vi "PING))) demo(not).vi"() -> ()   [LabVIEW 2016]
uses:
  <vilib>/myRIO/Instrument Drivers/Onboard IO/DIO/typedefs/DIO Reference.ctl
  <vilib>/myRIO/Common/Instrument Driver Framework/Utilities/typedefs/myRIO Generic Hardware Reference.ctl
  <vilib>/myRIO/Common/Instrument Driver Framework/Utilities/typedefs/Hardware Version Enum.ctl
  <vilib>/myRIO/Common/Instrument Driver Framework/Utilities/typedefs/myRIO v1.0 Reference.ctl
  <vilib>/myRIO/Common/Instrument Driver Framework/Utilities/typedefs/Generic FPGA Reference.ctl
  <vilib>/myRIO/Common/Instrument Driver Framework/myRIO v1.0/DIO/typedefs/DIO Channels List.ctl
  <vilib>/myRIO/Common/Instrument Driver Framework/myRIO v1.0/DIO/typedefs/DIO Channels Enum.ctl
  <vilib>/myRIO/Common/Instrument Driver Framework/myRIO v1.0/DIO/vis/myRIO v1.0 Close DIO.vi
  <vilib>/myRIO/Common/Instrument Driver Framework/myRIO v1.0/DIO/vis/myRIO v1.0 Unreserve DIO.vi
  <vilib>/myRIO/Common/Instrument Driver Framework/myRIO v1.0/DIO/vis/myRIO v1.0 Build MUX Configuration DIO.vi
  <vilib>/myRIO/Common/Instrument Driver Framework/myRIO v1.0/Resource Manager/vis/myRIO v1.0 Unreserve Channel List.vi
  <vilib>/myRIO/Common/Instrument Driver Framework/myRIO v1.0/Resource Manager/vis/myRIO v1.0 Create Configuration List.vi
  <vilib>/myRIO/Common/Instrument Driver Framework/myRIO v1.0/Resource Manager/vis/myRIO v1.0 Unreserve Channel.vi
  <vilib>/myRIO/Common/Instrument Driver Framework/myRIO v1.0/Resource Manager/vis/myRIO v1.0 Build Mutex Name.vi
  <vilib>/Utility/error.llb/Error Cluster From Error Code.vi
  <vilib>/myRIO/Common/Instrument Driver Framework/myRIO v1.0/DIO/vis/myRIO v1.0 Write DIO.vi
  <vilib>/myRIO/Common/Instrument Driver Framework/myRIO v1.0/DIO/vis/myRIO v1.0 Read DIO.vi
  <vilib>/myRIO/Common/Instrument Driver Framework/myRIO v1.0/DIO/vis/myRIO v1.0 Shutdown DIO.vi
  <vilib>/myRIO/Common/Instrument Driver Framework/myRIO v1.0/Resource Manager/vis/myRIO v1.0 Configure IO.vi
  <vilib>/myRIO/Common/Instrument Driver Framework/Utilities/vis/Configuration Manager.vi
  <vilib>/myRIO/Common/Instrument Driver Framework/Utilities/vis/IO Manager.vi
  <vilib>/myRIO/Common/Instrument Driver Framework/myRIO v1.0/myRIO v1.0 Close.vi
  <vilib>/myRIO/Instrument Drivers/Onboard IO/DIO/DIO.lvlib
panel:
  out "distance":u32
  in  "Channel Names":tag[](array[tag])
  out "Enum":T1(ring)
  in  "error in (no error)":errorcluster
  in  "stop":bool
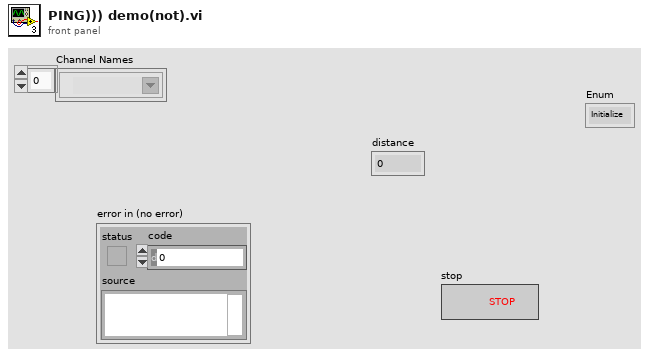
[diagram p1: front panel]
types:
  T1 = enum16{"Initialize", "Trigger pulse", "Wait pulse 1", "Wait pulse 2", "Calculate", "Stop"}
  T2 = typedef "DIO.lvlib/DIO Reference.ctl" = cluster{"myRIO Reference":T3, "DIO Channels List":T7}
  T3 = typedef "myRIO Generic Hardware Reference.ctl" = cluster{"myRIO Model":T4, "myRIO Hardware Reference":T5}
  T4 = typedef "Hardware Version Enum.ctl" = enum16{"Unknown", "myRIO-1900", "myRIO-1950", "roboRIO", "NI ELVIS RIO CM"}
  T5 = typedef "myRIO v1.0 Reference.ctl" = cluster{"Generic FPGA Reference":T6, "Allow multiple opens":bool}
  T6 = typedef "Generic FPGA Reference.ctl" = refnum<k20>
  T7 = typedef "DIO Channels List.ctl" = T8[]
  T8 = typedef "DIO Channels Enum.ctl" = enum16{"Not Connected", "C/DIO0", "C/DIO1", "C/DIO2", "C/DIO3", "C/DIO4", "C/DIO5", "C/DIO6", "C/DIO7", "A/DIO0", "A/DIO1", "A/DIO2", "A/DIO3", "A/DIO4", "A/DIO5", "A/DIO6", "A/DIO7", "A/DIO8", "A/DIO9", "A/DIO10", "A/DIO11", "A/DIO12", "A/DIO13", "A/DIO14", "A/DIO15", "B/DIO0", "B/DIO1", "B/DIO2", "B/DIO3", "B/DIO4", "B/DIO5", "B/DIO6", "B/DIO7", "B/DIO8", "B/DIO9", "B/DIO10", "B/DIO11", "B/DIO12", "B/DIO13", "B/DIO14", "B/DIO15", "LED0", "LED1", "LED2", "LED3", "Button0", "DIO/DIO0", "DIO/DIO1", "DIO/DIO2", "DIO/DIO3", "DIO/DIO4", "DIO/DIO5", "DIO/DIO6", "DIO/DIO7", "DIO/DIO8", "DIO/DIO9", "SPI/CS0", "SPI/CS1", "SPI/CS2", "SPI/CS3", "LED RADIO (Green)", "LED RADIO (Red)", "LED COMM (Green)", "LED COMM (Red)", "LED MODE (Green)", "LED MODE (Red)"}
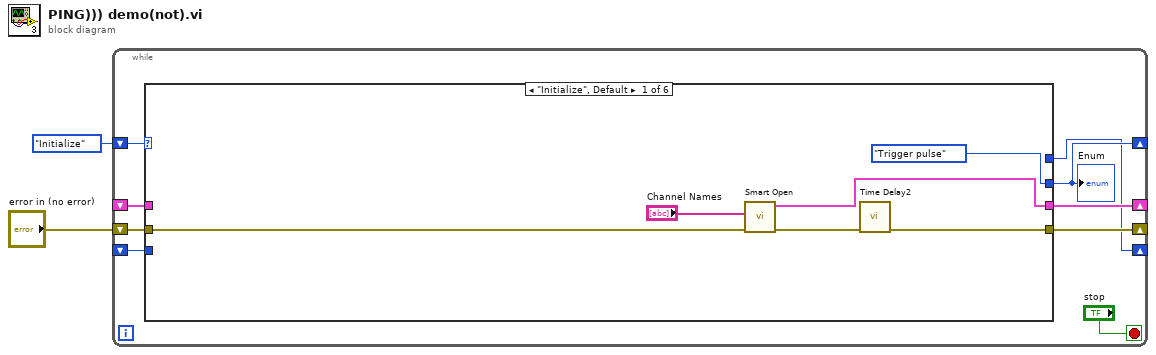
[diagram p0: block diagram]
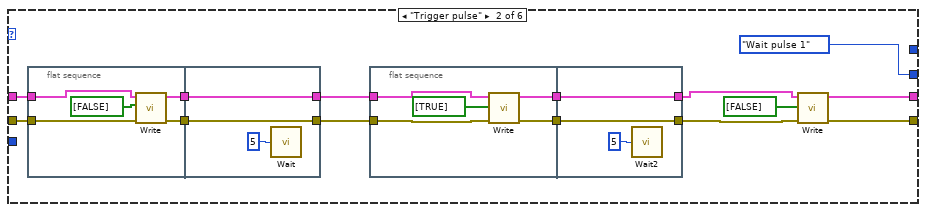
[diagram p2: hidden frame]
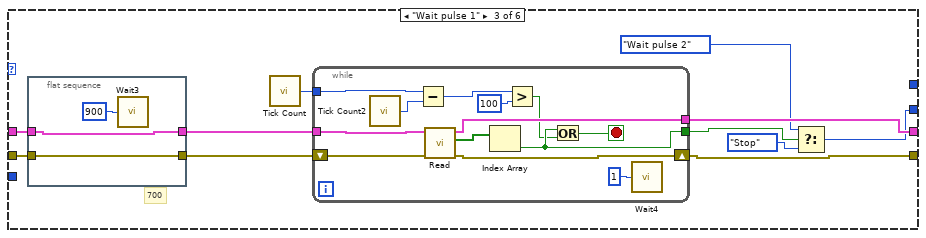
[diagram p3: hidden frame]
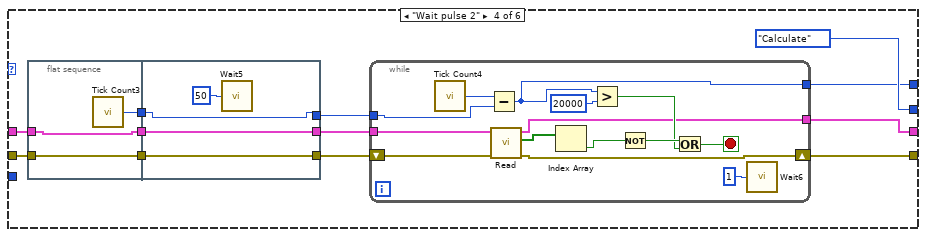
[diagram p4: hidden frame]
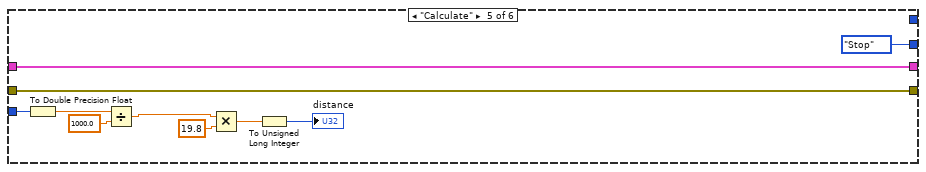
[diagram p5: hidden frame]
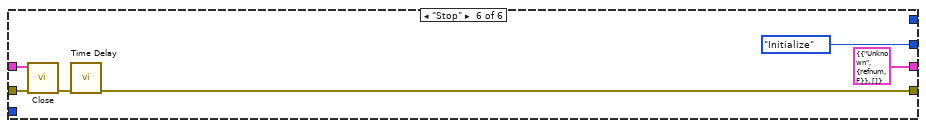
[diagram p6: hidden frame]
diagram:
  n1 = while {
    shift-right: [w9] -> _
    shift-left: T1."Initialize" -> [w10]
    shift-right: [w7] -> _
    shift-left: _ -> [w6]
    shift-right: [w5] -> _
    shift-left: "error in (no error)" -> [w8]
    shift-right: [w3] -> _
    shift-left: _ -> [w4]
    stop <- "stop" stop-if-true
    n2 = case shown="\"Initialize\", Default" w10 {
      tunnel: [T1."Trigger pulse" T1."Wait pulse 1" w49 T1."Calculate" T1."Stop" T1."Initialize"] -> w9
      tunnel: w8 -> [w16 w29 w57 w78 w112 w121]
      tunnel: [w15 w19 w54 w75 w113 T2 {"myRIO Reference"={"myRIO Model"=enum."Unknown", "myRIO Hardware Reference"={"Generic FPGA Reference"=refnum, "Allow multiple opens"=FALSE}}, "DIO Channels List"=[]} ("DIO Ref Out")] -> w7
      tunnel: w6 -> [_ w26 w55 w81 w113 w122]
      tunnel: [w12 w18 w53 w76 w112 w118] -> w5
      tunnel: w4 -> [_ _ _ _ w114 _]
      tunnel: [_ _ _ w77 _ _] -> w3
      frame "Initialize", Default {
        n3 = call <vilib>:"Smart Open.vi"("error in (no error)"=w16, "Channel Names"="Channel Names") -> ("error out"=w14:errorcluster, "DIO Ref Out"=w15:T2)  [unwired: 8 in]
        n4 = call "Time Delay2"("error in (no error)"=w14) -> ("error out"=w12:errorcluster)  [unwired: 10 in]
      }
      frame "Trigger pulse" {
        n5 = flat-sequence {
          tunnel: w29 -> [w43]
          tunnel: [w42] -> w27
          tunnel: w26 -> [w41]
          tunnel: [w40] -> w24
          tunnel: [w46] -> w28
          tunnel: w27 -> [w46]
          tunnel: [w45] -> w25
          tunnel: w24 -> [w45]
          frame #0 {
            n6 = call <vilib>:"Write.vi"("error in (no error)"=w43, "Values"=bool[] [FALSE], "DIO Ref In"=w41) -> ("error out"=w42:errorcluster, "DIO Ref Out"=w40:T2)  [unwired: 6 in]
          }
          frame #1 {
            n7 = call "Wait"("Count(uSec)"=u32 5) -> ()  [unwired: 1 out]
          }
        }
        n8 = flat-sequence {
          tunnel: w28 -> [w35]
          tunnel: w25 -> [w34]
          tunnel: [w33] -> w23
          tunnel: [w32] -> w21
          tunnel: w23 -> [w38]
          tunnel: [w38] -> w22
          tunnel: w21 -> [w37]
          tunnel: [w37] -> w20
          frame #0 {
            n9 = call <vilib>:"Write.vi"("error in (no error)"=w35, "Values"=bool[] [TRUE], "DIO Ref In"=w34) -> ("error out"=w32:errorcluster, "DIO Ref Out"=w33:T2)  [unwired: 6 in]
          }
          frame #1 {
            n10 = call "Wait2"("Count(uSec)"=u32 5) -> ()  [unwired: 1 out]
          }
        }
        n11 = call <vilib>:"Write.vi"("error in (no error)"=w20, "Values"=bool[] [FALSE], "DIO Ref In"=w22) -> ("error out"=w18:errorcluster, "DIO Ref Out"=w19:T2)  [unwired: 6 in]
      }
      frame "Wait pulse 1" {
        # "700"
        n12 = flat-sequence {
          tunnel: [w73] -> w58
          tunnel: w57 -> [w73]
          tunnel: [w72] -> w56
          tunnel: w55 -> [w72]
          frame #0 {
            n13 = call "Wait3"("Count(uSec)"=u32 900) -> ()  [unwired: 1 out]
          }
        }
        n14 = call "Tick Count"() -> ("Tick Count(uSec)"=w52:u32)
        n15 = while {
          tunnel: w56 -> [w70]
          tunnel: [w69] -> w54
          shift-right: [w66] -> w53
          shift-left: w58 -> [w71]
          tunnel: w52 -> [w61]
          tunnel: [w60] -> w48
          stop <- w67 stop-if-true
          n16 = call "Tick Count2"() -> ("Tick Count(uSec)"=w62:u32)
          n17 = Subtract(x=w61, y=w62) -> (x-y=w63:u32)
          n18 = call <vilib>:"Read.vi"("error in (no error)"=w71, "DIO Ref In"=w70) -> ("error out"=w66:errorcluster, "Values"=w68:bool[], "DIO Ref Out"=w69:T2)  [unwired: 7 in]
          n19 = Index Array(array=w68) -> (element=w60:bool)  [unwired: 1 in]
          n20 = Greater?(x=w63, y=u32 100) -> (0:w59:bool)
          n21 = Or(x=w60, y=w59) -> (x .or. y?=w67:bool)
          n22 = call "Wait4"("Count(uSec)"=u32 1) -> ()  [unwired: 1 out]
        }
        n23 = Select(t=T1."Wait pulse 2", s=w48, f=T1."Stop") -> (s? t:f=w49:T1)
      }
      frame "Wait pulse 2" {
        n24 = flat-sequence {
          tunnel: [w103] -> w84
          tunnel: [w102] -> w82
          tunnel: w81 -> [w102]
          tunnel: [w101] -> w79
          tunnel: w78 -> [w101]
          tunnel: [w106] -> w85
          tunnel: w84 -> [w106]
          tunnel: [w105] -> w83
          tunnel: w82 -> [w105]
          tunnel: [w104] -> w80
          tunnel: w79 -> [w104]
          frame #0 {
            n25 = call "Tick Count3"() -> ("Tick Count(uSec)"=w103:u32)
          }
          frame #1 {
            n26 = call "Wait5"("Count(uSec)"=u32 50) -> ()  [unwired: 1 out]
          }
        }
        n27 = while {
          tunnel: w85 -> [w88]
          tunnel: w83 -> [w100]
          tunnel: [w92] -> w77
          tunnel: [w89] -> w75
          shift-right: [w90] -> w76
          shift-left: w80 -> [w99]
          stop <- w95 stop-if-true
          n28 = call "Tick Count4"() -> ("Tick Count(uSec)"=w87:u32)
          n29 = Subtract(x=w87, y=w88) -> (x-y=w92:u32)
          n30 = call <vilib>:"Read.vi"("error in (no error)"=w99, "DIO Ref In"=w100) -> ("error out"=w90:errorcluster, "Values"=w98:bool[], "DIO Ref Out"=w89:T2)  [unwired: 7 in]
          n31 = Index Array(array=w98) -> (element=w96:bool)  [unwired: 1 in]
          n32 = Greater?(x=w92, y=u32 20000) -> (0:w94:bool)
          n33 = Not(x=w96) -> (.not. x?=w97:bool)
          n34 = Or(x=w97, y=w94) -> (x .or. y?=w95:bool)
          n35 = call "Wait6"("Count(uSec)"=u32 1) -> ()  [unwired: 1 out]
        }
      }
      frame "Calculate" {
        n36 = To Double Precision Float(number=w114) -> (double precision float=w116:dbl)
        n37 = Divide(x=w116, y=1000.0) -> (x/y=w110:dbl)
        n38 = Multiply(x=w110, y=19.8) -> (x*y=w109:dbl)
        n39 = To Unsigned Long Integer(number=w109) -> (unsigned 32bit integer=→"distance":u32)
      }
      frame "Stop" {
        n40 = call <vilib>:"Close.vi"("error in (no error)"=w121, "DIO Ref In"=w122) -> ("error out"=w119:errorcluster)  [unwired: 9 in]
        n41 = call "Time Delay"("error in (no error)"=w119) -> ("error out"=w118:errorcluster)  [unwired: 10 in]
      }
    }
    "Enum" <- w9
  }
